vi "Main.vi"() -> ()   [LabVIEW 2021]
doc: "This template is for the Queued Message Handler design pattern.\n\nThe Event Handling Loop generates messages based on user interface actions.\n\nThe Message Handling Loop processes messages generated by the Event Handling Loop, or by other messages. The messages are string values, so new messages can be added easily to the Message Cases case structure in the Message Handling Loop. Each message cluster can also provide an optional value for Message Data, which is a variant that can be converted to whatever message-specific data is required."
uses:
  Controls/UI Data.ctl
  support/Message Queue/Message Queue.lvlib
  <vilib>/Utility/error.llb/Error Cluster From Error Code.vi
  support/User Event - Stop/User Event - Stop.lvlib
  support/Message Queue/Enqueue Message (Single).vi
  <vilib>/ErrorRing/Error Ring.xnode
  Controls/Status Lights.ctl
panel:
  in  "Start Pressure Logging":bool
  out "Speed Indicator":dbl
  in  "Release Brake":bool
  in  "Retract":bool
  out "Status":T1
  in  "Speed (v)":dbl(knob) scale=0.0..5.0
  out "Status":string
  in  "Extend":bool
  in  "Apply Brake":bool
  in  "Exit":bool
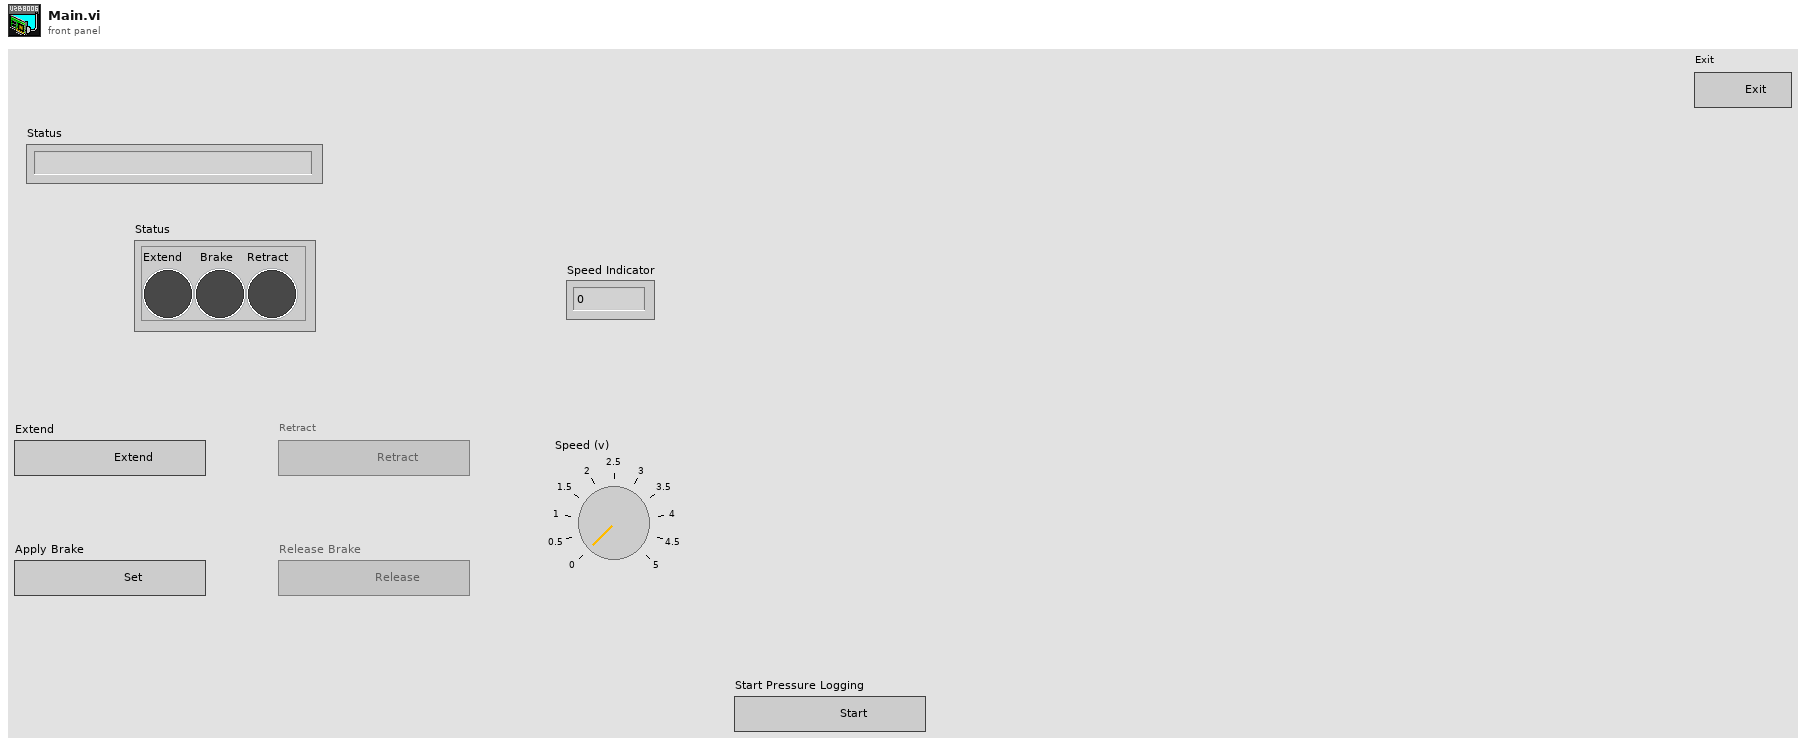
[diagram p1: front panel]
types:
  T1 = typedef "Status Lights.ctl" = cluster{"Extend":bool, "Brake":bool, "Retract":bool}
  T2 = typedef "UI Data.ctl" = cluster{"Boolean":bool, "String":string, "Speed":dbl, "Apply Brake Ref":refnum<vi>, "Release Brake Ref":refnum<vi>, "Extend Ref":refnum<vi>, "Retract Ref":refnum<vi>, "Data Display Ref":refnum<vi>, "Exit Button Ref":refnum<vi>, "Status":T1, "Pressure Ref":refnum<vi>}
  T3 = typedef "Message Queue.lvlib/All Message Queues.ctl" = cluster{"UI":refnum<queue>}
  T4 = typedef "DAQ Refnums.ctl" = cluster{"Direction Ref":refnum<k21>, "Brake Ref":refnum<k21>, "Speed Ref":refnum<k21>, "Pressure Ref":refnum<k21>}
  T5 = enum8{"Enabled", "Disabled", "Disabled and Grayed Out"}
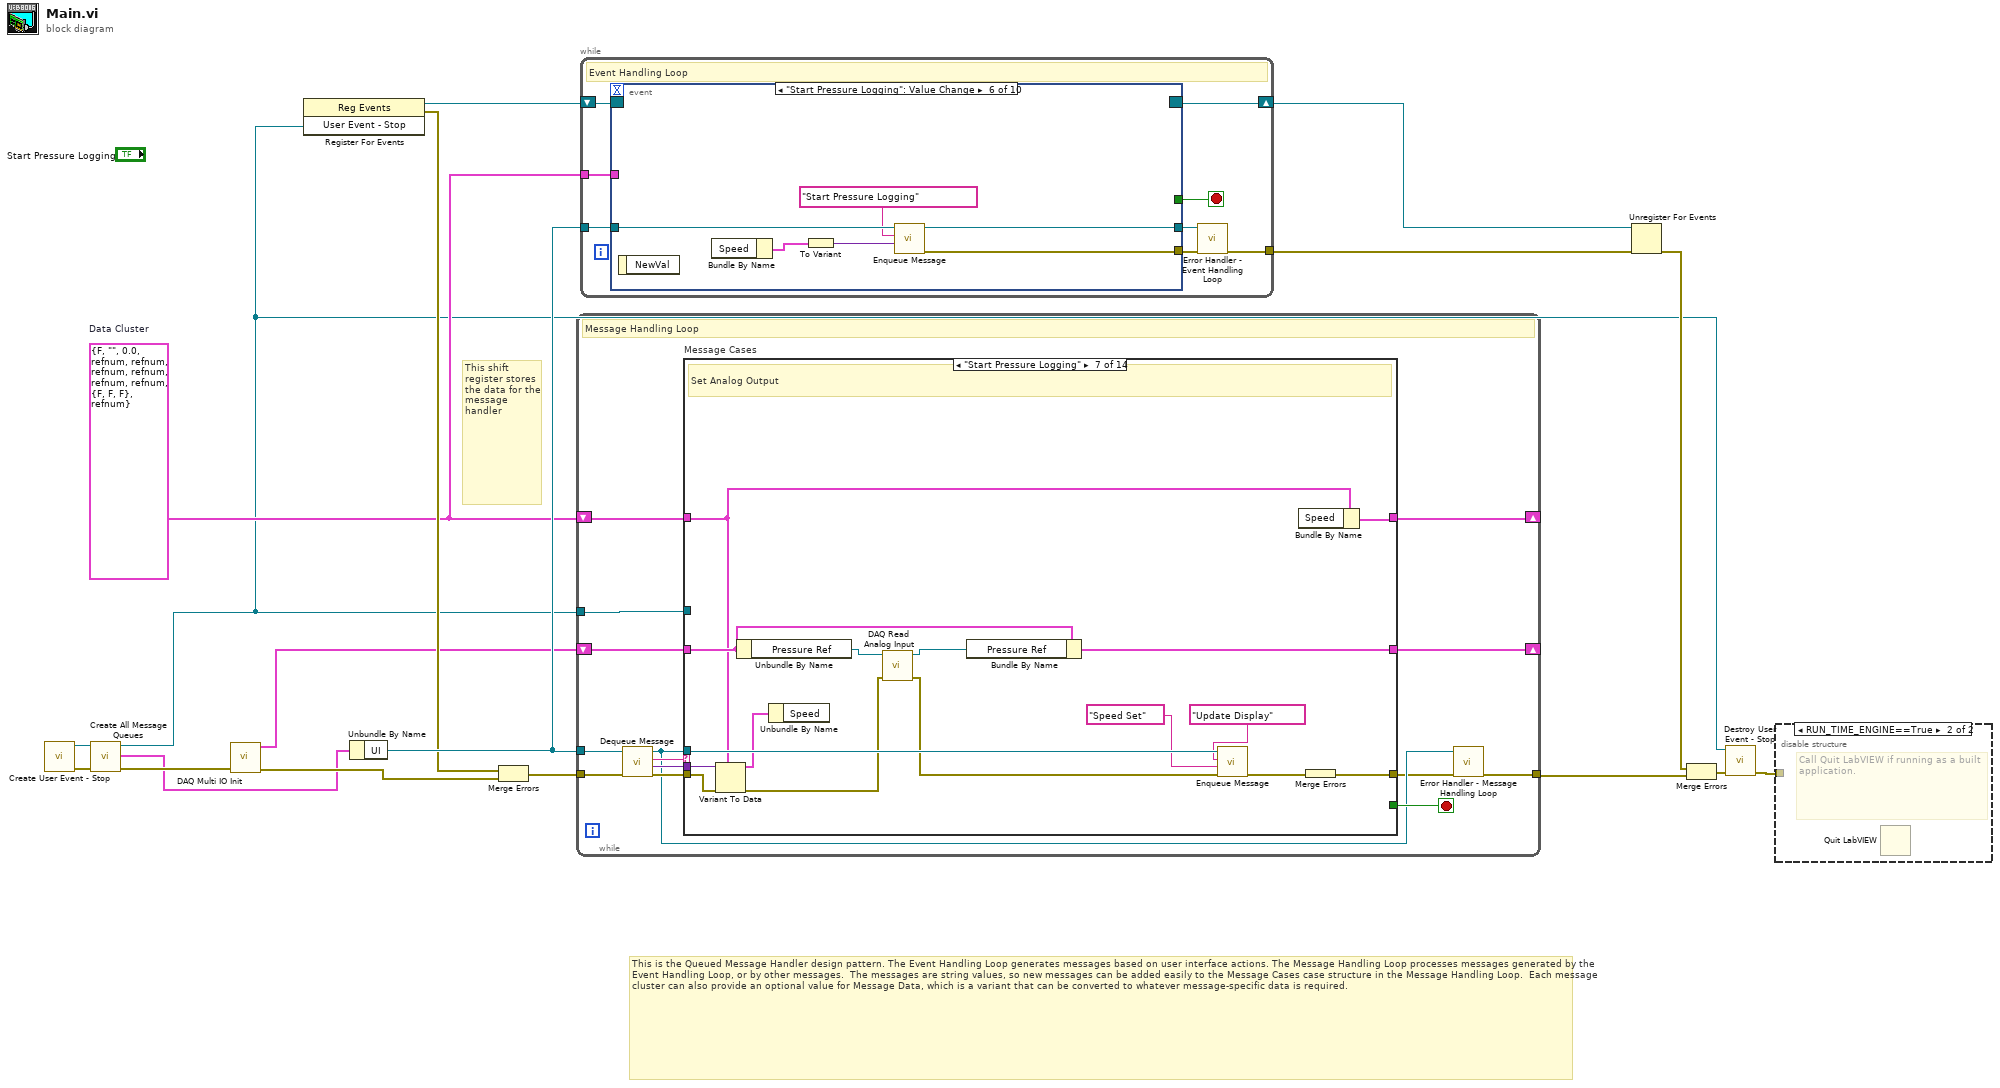
[diagram p0: block diagram]
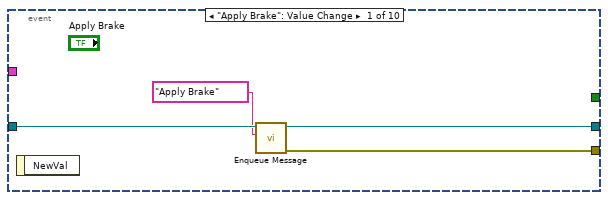
[diagram p3: hidden frame]
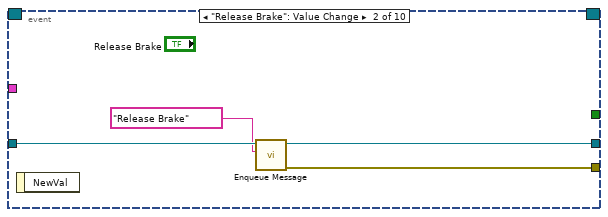
[diagram p4: hidden frame]
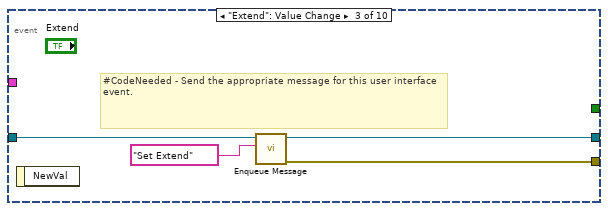
[diagram p5: hidden frame]
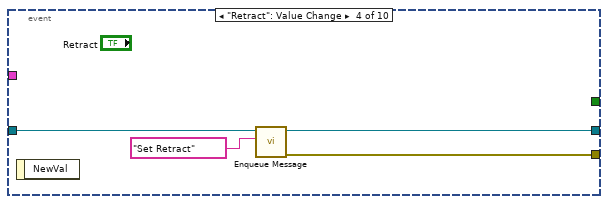
[diagram p6: hidden frame]
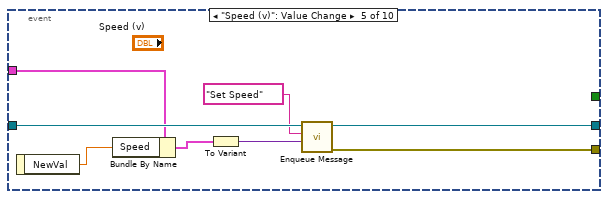
[diagram p7: hidden frame]
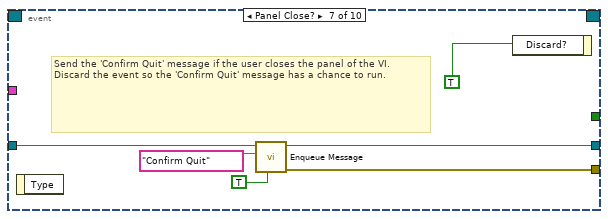
[diagram p8: hidden frame]
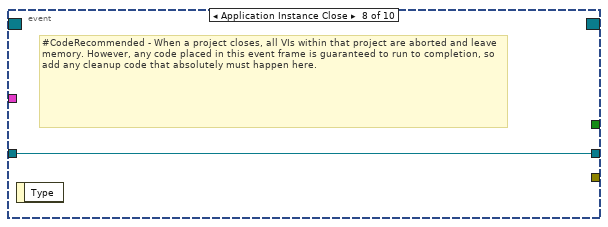
[diagram p9: hidden frame]
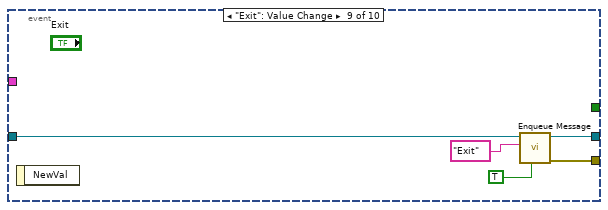
[diagram p10: hidden frame]
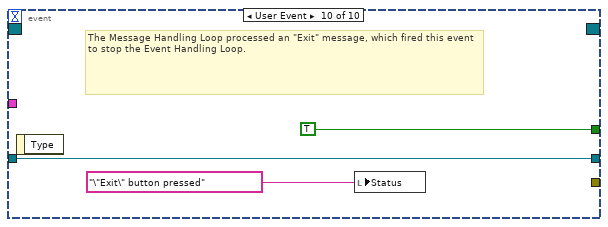
[diagram p11: hidden frame]
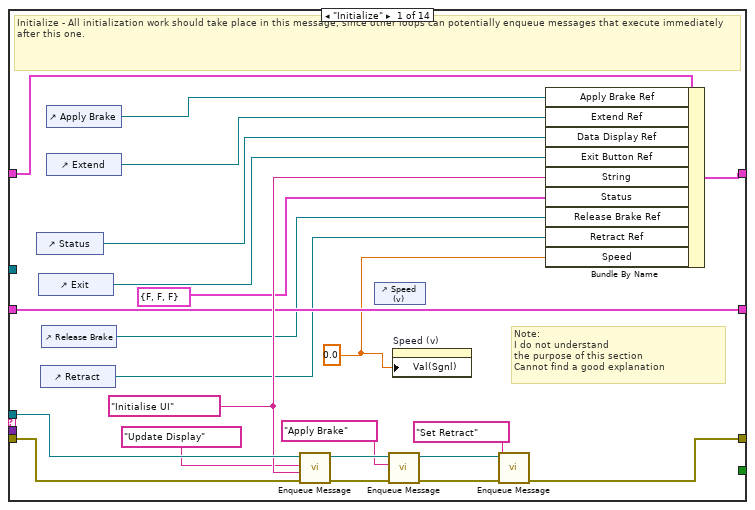
[diagram p12: hidden frame]
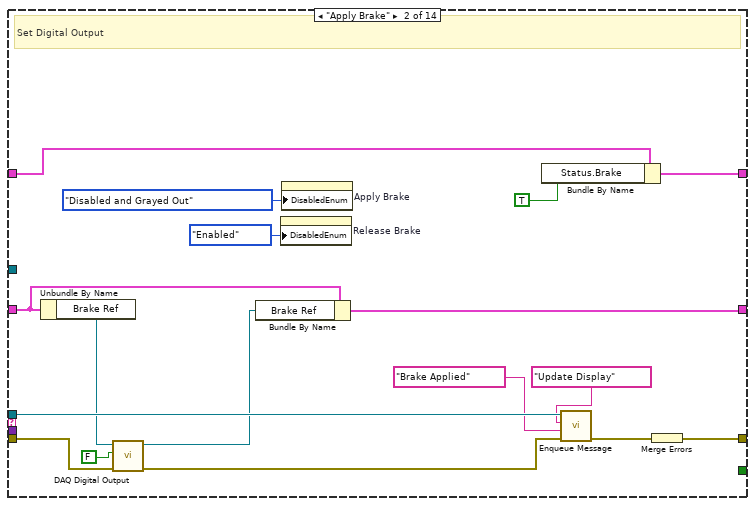
[diagram p13: hidden frame]
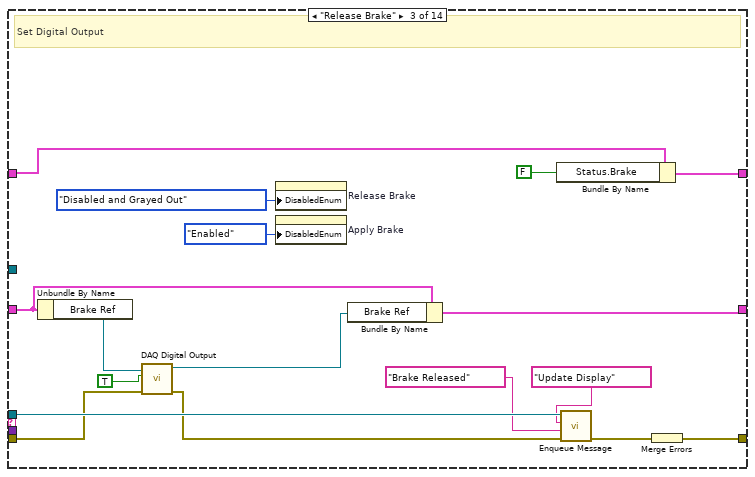
[diagram p14: hidden frame]
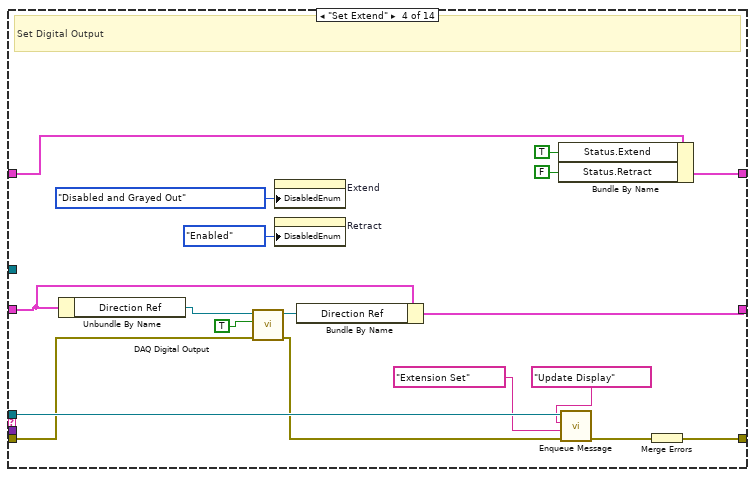
[diagram p15: hidden frame]
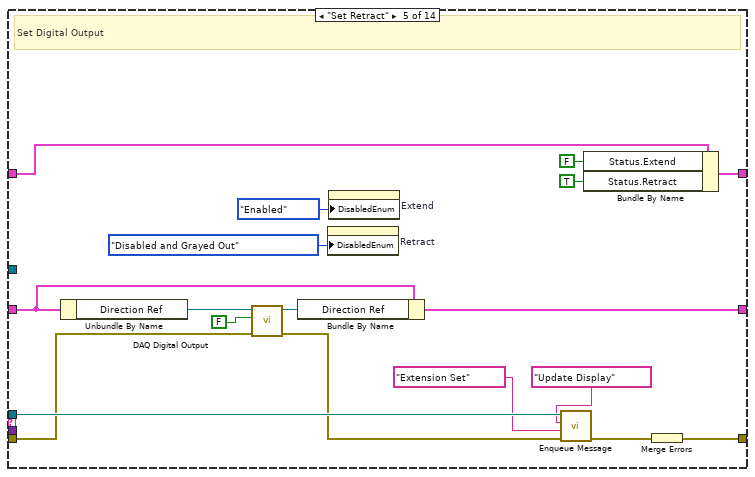
[diagram p16: hidden frame]
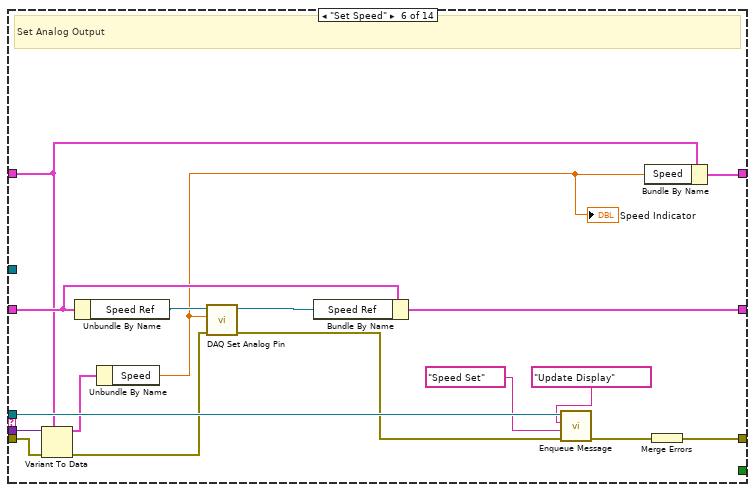
[diagram p17: hidden frame]
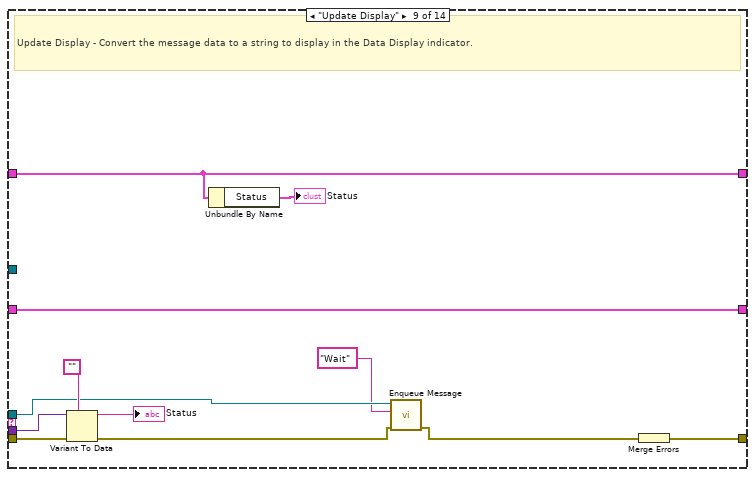
[diagram p19: hidden frame]
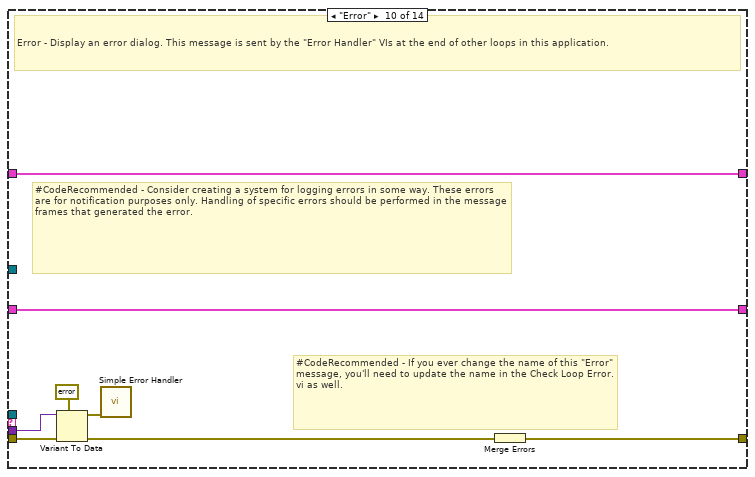
[diagram p20: hidden frame]
diagram:
  w5 = T2 {"Boolean"=FALSE, "String"="", "Speed"=0.0, "Apply Brake Ref"=refnum, "Release Brake Ref"=refnum, "Extend Ref"=refnum, "Retract Ref"=refnum, "Data Display Ref"=refnum, "Exit Button Ref"=refnum, "Status"={"Extend"=FALSE, "Brake"=FALSE, "Retract"=FALSE}, "Pressure Ref"=refnum}  # Data Cluster
  # "This is the Queued Message Handler design pattern. The Event Handling Loop generates messages based on user interface actions. The Message Handling Loop processes messages generated by the Event Handling Loop, or by other messages.  The messages are string values, so new messages can be added easily to the Message Cases case structure in the Message Handling Loop.  Each message cluster can also provide an optional value for Message Data, which is a variant that can be converted to whatever message-specific data is required."
  # "This shift register stores the data for the message handler"
  n1 = call "Create User Event - Stop.vi"() -> ("error out"=w16:errorcluster, "User Event - Stop"=w4:refnum<user-event>)  [unwired: 10 in]
  n2 = call "Create All Message Queues.vi"("error in (no error)"=w16) -> ("error out"=w3:errorcluster, "Message Queues out"=w1:T3)  [unwired: 9 in]
  n3 = call "DAQ Multi IO Init.vi"("error in"=w3) -> ("error out"=w2:errorcluster, "DAQ Ref Cluster"=w6:T4)  [unwired: 9 in]
  n4 = register-events(w4) -> (reference out=w10:refnum<event-registration>, error out=w9:errorcluster)  [unwired: 2 in]
  n5 = Unbundle By Name(w1) -> ("UI"=w17:refnum<queue>)
  n6 = Merge Errors(w9, w2) -> (w7:errorcluster)
  n7 = while {
    tunnel: w17 -> [w25]
    shift-right: [w20] -> _
    shift-left: w5 -> [w31]
    tunnel: w4 -> [w29]
    tunnel: [w23] -> w8
    tunnel: w7 -> [w21]
    shift-right: [w18] -> _
    shift-left: w6 -> [w19]
    stop <- w30 stop-if-true
    # "Message Handling Loop"
    n8 = call "Dequeue Message.vi"("error in (no error)"=w21, "Message Queue"=w25) -> ("error out"=w28:errorcluster, "Message Data"=w26:variant, "Message"=w27:string, "dup Message Queue"=w24:refnum<queue>)  [unwired: 6 in]
    n9 = case "Message Cases" shown="\"Start Pressure Logging\"" w27 {
      selector: w27 -> [_ _ _ _ _ _ _ _ _ _ _ _ _ w215]
      tunnel: w24 -> [w49 w68 w85 w103 w121 w138 w154 _ w162 _ w183 _ w213 _]
      tunnel: w28 -> [w53 w66 w83 w101 w119 w129 w148 w158 w170 w179 w187 w191 w208 _]
      tunnel: [w34 w70 w87 w105 w123 w140 w156 w158 w171 w173 w185 w189 w210 w216] -> w22
      tunnel: w31 -> [w41 w60 w71 w88 w108 w126 w146 w159 w166 w178 w186 w190 w212 w217]
      tunnel: [w52 w63 w80 w98 w116 w125 w145 w159 w166 w178 w186 w190 w212 w217] -> w20
      tunnel: [_ _ _ _ _ _ _ _ _ _ _ _ TRUE _] -> w30
      tunnel: w26 -> [_ _ _ _ _ w130 w149 _ w169 w177 _ _ w205 _]
      tunnel: w29 -> [_ _ _ _ _ _ _ _ _ _ _ _ w209 _]
      tunnel: w19 -> [w45 w58 w75 w94 w112 w135 w151 w157 w160 w172 w180 w188 w197 w214]
      tunnel: [w45 w57 w74 w93 w111 w134 w150 w157 w160 w172 w180 w188 w198 w214] -> w18
      frame "Initialize" {
        w42 = 0.0 ("Speed")
        w48 = "Initialise UI" ("Initial Message")
        # "Note:\nI do not understand\nthe purpose of this section\nCannot find a good explanation"
        # "Initialize - All initialization work should take place in this message, since other loops can potentially enqueue messages that execute immediately after this one."
        n10 = control-ref of="Status"() -> (w51:refnum<vi>)
        n11 = control-ref of="Exit"() -> (w50:refnum<vi>)
        n12 = control-ref of="Retract"() -> (w43:refnum<vi>)
        n13 = control-ref of="Release Brake"() -> (w44:refnum<vi>)
        n14 = control-ref of="Apply Brake"() -> (w47:refnum<vi>)
        n15 = control-ref of="Extend"() -> (w40:refnum<vi>)
        n16 = call-poly "Enqueue Message.vi"("error in (no error)"=w53, "Message Data"=w48, "Message"="Update Display", "Message Queue"=w49) -> ("error out"=w38:errorcluster, "dup Message Queue"=w37:refnum<queue>)  [unwired: 6 in]
        n17 = control-ref of="Speed (v)"() -> ()  [unwired: 1 out]
        n18 = call-poly "Enqueue Message.vi"("error in (no error)"=w38, "Message"="Apply Brake", "Message Queue"=w37) -> ("error out"=w35:errorcluster, "dup Message Queue"=w33:refnum<queue>)  [unwired: 7 in]
        n19 = property on="Speed (v)" class="Knob (strict)"("Val(Sgnl)"=w42) -> ()  [unwired: 2 in, 2 out]
        n20 = call-poly "Enqueue Message.vi"("error in (no error)"=w35, "Message"="Set Retract", "Message Queue"=w33) -> ("error out"=w34:errorcluster)  [unwired: 7 in, 1 out]
        n21 = Bundle By Name(cluster=w41, "Apply Brake Ref"=w47, "Extend Ref"=w40, "Data Display Ref"=w51, "Exit Button Ref"=w50, "String"=w48, "Status"=T1 {"Extend"=FALSE, "Brake"=FALSE, "Retract"=FALSE}, "Release Brake Ref"=w44, "Retract Ref"=w43, "Speed"=w42) -> (w52:T2)
      }
      frame "Apply Brake" {
        # "Set Digital Output"
        n22 = Unbundle By Name(w58) -> ("Brake Ref"=w59:refnum<k21>)
        n23 = call "DAQ Digital Output.vi"("error in"=w66, "data"=FALSE, "task/channels in"=w59) -> ("error out"=w65:errorcluster, "task out"=w56:refnum<k21>)  [unwired: 6 in, 1 out]
        n24 = Bundle By Name(cluster=w58, "Brake Ref"=w56) -> (w57:T4)
        n25 = property on="Release Brake" class="Bool"("DisabledEnum"=T5."Enabled" ("Disabled")) -> ()  [unwired: 2 in, 2 out]
        n26 = property on="Apply Brake" class="Bool"("DisabledEnum"=T5."Disabled and Grayed Out" ("Disabled")) -> ()  [unwired: 2 in, 2 out]
        n27 = Bundle By Name(cluster=w60, "Status.Brake"=TRUE) -> (w63:T2)
        n28 = call-poly "Enqueue Message.vi"("error in (no error)"=w65, "Message Data"="Brake Applied" ("\"Do Something\" button pressed"), "Message"="Update Display", "Message Queue"=w68) -> ("error out"=w69:errorcluster)  [unwired: 6 in, 1 out]
        n29 = Merge Errors(w69) -> (w70:errorcluster)
      }
      frame "Release Brake" {
        # "Set Digital Output"
        n30 = Unbundle By Name(w75) -> ("Brake Ref"=w77:refnum<k21>)
        n31 = call "DAQ Digital Output.vi"("error in"=w83, "data"=TRUE, "task/channels in"=w77) -> ("error out"=w82:errorcluster, "task out"=w76:refnum<k21>)  [unwired: 6 in, 1 out]
        n32 = property on="Release Brake" class="Bool"("DisabledEnum"=T5."Disabled and Grayed Out" ("Disabled")) -> ()  [unwired: 2 in, 2 out]
        n33 = property on="Apply Brake" class="Bool"("DisabledEnum"=T5."Enabled" ("Disabled")) -> ()  [unwired: 2 in, 2 out]
        n34 = Bundle By Name(cluster=w75, "Brake Ref"=w76) -> (w74:T4)
        n35 = Bundle By Name(cluster=w71, "Status.Brake"=FALSE ("Boolean")) -> (w80:T2)
        n36 = call-poly "Enqueue Message.vi"("error in (no error)"=w82, "Message Data"="Brake Released" ("\"Do Something\" button pressed"), "Message"="Update Display", "Message Queue"=w85) -> ("error out"=w86:errorcluster)  [unwired: 6 in, 1 out]
        n37 = Merge Errors(w86) -> (w87:errorcluster)
      }
      frame "Set Extend" {
        # "Set Digital Output"
        n38 = Unbundle By Name(w94) -> ("Direction Ref"=w96:refnum<k21>)
        n39 = call "DAQ Digital Output.vi"("error in"=w101, "data"=TRUE, "task/channels in"=w96) -> ("error out"=w100:errorcluster, "task out"=w95:refnum<k21>)  [unwired: 6 in, 1 out]
        n40 = property on="Extend" class="Bool"("DisabledEnum"=T5."Disabled and Grayed Out" ("Disabled")) -> ()  [unwired: 2 in, 2 out]
        n41 = property on="Retract" class="Bool"("DisabledEnum"=T5."Enabled" ("Disabled")) -> ()  [unwired: 2 in, 2 out]
        n42 = Bundle By Name(cluster=w94, "Direction Ref"=w95) -> (w93:T4)
        n43 = Bundle By Name(cluster=w88, "Status.Extend"=TRUE ("Status.Retract"), "Status.Retract"=FALSE ("Status.Extend")) -> (w98:T2)
        n44 = call-poly "Enqueue Message.vi"("error in (no error)"=w100, "Message Data"="Extension Set" ("\"Do Something\" button pressed"), "Message"="Update Display", "Message Queue"=w103) -> ("error out"=w104:errorcluster)  [unwired: 6 in, 1 out]
        n45 = Merge Errors(w104) -> (w105:errorcluster)
      }
      frame "Set Retract" {
        # "Set Digital Output"
        n46 = Unbundle By Name(w112) -> ("Direction Ref"=w114:refnum<k21>)
        n47 = call "DAQ Digital Output.vi"("error in"=w119, "data"=FALSE, "task/channels in"=w114) -> ("error out"=w118:errorcluster, "task out"=w113:refnum<k21>)  [unwired: 6 in, 1 out]
        n48 = Bundle By Name(cluster=w112, "Direction Ref"=w113) -> (w111:T4)
        n49 = property on="Retract" class="Bool"("DisabledEnum"=T5."Disabled and Grayed Out" ("Disabled")) -> ()  [unwired: 2 in, 2 out]
        n50 = property on="Extend" class="Bool"("DisabledEnum"=T5."Enabled" ("Disabled")) -> ()  [unwired: 2 in, 2 out]
        n51 = call-poly "Enqueue Message.vi"("error in (no error)"=w118, "Message Data"="Extension Set" ("\"Do Something\" button pressed"), "Message"="Update Display", "Message Queue"=w121) -> ("error out"=w122:errorcluster)  [unwired: 6 in, 1 out]
        n52 = Bundle By Name(cluster=w108, "Status.Extend"=FALSE ("Status.Retract"), "Status.Retract"=TRUE ("Status.Extend")) -> (w116:T2)
        n53 = Merge Errors(w122) -> (w123:errorcluster)
      }
      frame "Set Speed" {
        # "Set Analog Output"
        n54 = Variant To Data(error in=w129, type=w126, Variant=w130) -> (data=w127:T2, error out=w128:errorcluster)
        n55 = Unbundle By Name(w135) -> ("Speed Ref"=w133:refnum<k21>)
        n56 = Unbundle By Name(w127) -> ("Speed"=w124:dbl)
        "Speed Indicator" <- w124
        n57 = call "DAQ Set Analog Pin.vi"("error in"=w128, "Voltage"=w124, "task/channels in"=w133) -> ("error out"=w131:errorcluster, "task out"=w132:refnum<k21>)  [unwired: 6 in, 1 out]
        n58 = Bundle By Name(cluster=w135, "Speed Ref"=w132) -> (w134:T4)
        n59 = call-poly "Enqueue Message.vi"("error in (no error)"=w131, "Message Data"="Speed Set" ("\"Do Something\" button pressed"), "Message"="Update Display", "Message Queue"=w138) -> ("error out"=w139:errorcluster)  [unwired: 6 in, 1 out]
        n60 = Bundle By Name(cluster=w126, "Speed"=w124) -> (w125:T2)
        n61 = Merge Errors(w139) -> (w140:errorcluster)
      }
      frame "Start Pressure Logging" {
        # "Set Analog Output"
        n62 = Variant To Data(error in=w148, type=w146, Variant=w149) -> (data=w147:T2, error out=w143:errorcluster)
        n63 = Unbundle By Name(w151) -> ("Pressure Ref"=w144:refnum<k21>)
        n64 = Unbundle By Name(w147) -> ()  [unwired: 1 out]
        n65 = call "DAQ Read Analog Input.vi"("error in"=w143, "task/channels in"=w144) -> ("error out"=w142:errorcluster, "task out"=w141:refnum<k21>)  [unwired: 7 in, 1 out]
        n66 = Bundle By Name(cluster=w151, "Pressure Ref"=w141) -> (w150:T4)
        n67 = call-poly "Enqueue Message.vi"("error in (no error)"=w142, "Message Data"="Speed Set" ("\"Do Something\" button pressed"), "Message"="Update Display", "Message Queue"=w154) -> ("error out"=w155:errorcluster)  [unwired: 6 in, 1 out]
        n68 = Bundle By Name(cluster=w146) -> (w145:T2)  [unwired: 1 in]
        n69 = Merge Errors(w155) -> (w156:errorcluster)
      }
      frame "Wait" {
        # "Wait case - wait for user input"
      }
      frame "Update Display" {
        # "Update Display - Convert the message data to a string to display in the Data Display indicator."
        n70 = Variant To Data(error in=w170, type="", Variant=w169) -> (data=→"Status":string, error out=w164:errorcluster)
        n71 = Unbundle By Name(w166) -> ("Status"=→"Status":T1)
        n72 = call-poly "Enqueue Message.vi"("error in (no error)"=w164, "Message"="Wait", "Message Queue"=w162) -> ("error out"=w163:errorcluster)  [unwired: 7 in, 1 out]
        n73 = Merge Errors(w163) -> (w171:errorcluster)
      }
      frame "Error" {
        # "#CodeRecommended - If you ever change the name of this \"Error\" message, you'll need to update the name in the Check Loop Error.vi as well."
        # "#CodeRecommended - Consider creating a system for logging errors in some way. These errors are for notification purposes only. Handling of specific errors should be performed in the message frames that generated the error."
        # "Error - Display an error dialog. This message is sent by the \"Error Handler\" VIs at the end of other loops in this application."
        n74 = Variant To Data(error in=w179, type=errorcluster {"status"=FALSE, "code"=0, "source"=""} ("error constant"), Variant=w177) -> (data=w175:errorcluster, error out=w174:errorcluster)
        n75 = call <vilib>:"Simple Error Handler.vi"("error in (no error)"=w175) -> ()  [unwired: 4 in, 5 out]
        n76 = Merge Errors(w174) -> (w173:errorcluster)
      }
      frame "Confirm Quit" {
        # "#CodeNeeded - If you want to provide an \"Are you sure\" dialog (or some other notification) before the application exits, place that code here. This message is typically sent from a Panel Close? event."
        # "Confirm Quit - Message that can confirm whether or not the user wants to exit the application."
        n77 = call-poly "Enqueue Message.vi"("Priority Message? (F)"=TRUE, "error in (no error)"=w187, "Message"="Exit", "Message Queue"=w183) -> ("error out"=w184:errorcluster)  [unwired: 6 in, 1 out]
        n78 = Merge Errors(w184) -> (w185:errorcluster)
      }
      frame "---Copy This Frame---" {
        # "Duplicate this frame when creating new messages.  Change this comment in the duplicated frame to describe this message."
        n79 = Merge Errors(w191) -> (w189:errorcluster)
      }
      frame "Exit" {
        # "Stop the VI"
        # "Release the message queue reference"
        # "Exit - Exit the application."
        n80 = Release Queue(queue=w213, error in (no error)=w208) -> (error out=w204:errorcluster)  [unwired: 1 in, 2 out]
        n81 = call "Fire User Event - Stop.vi"("User Event - Stop"=w209) -> ("error out"=w193:errorcluster)  [unwired: 10 in]
        n82 = Variant To Data(type=errorcluster {"status"=FALSE, "code"=0, "source"=""} ("error constant"), Variant=w205) -> (data=w206:errorcluster)  [unwired: 1 in, 1 out]
        n83 = Unbundle By Name(w197) -> ("Direction Ref"=w201:refnum<k21>, "Brake Ref"=w200:refnum<k21>, "Speed Ref"=w199:refnum<k21>)
        n84 = call <vilib>:"Simple Error Handler.vi"("error in (no error)"=w206) -> ()  [unwired: 4 in, 5 out]
        n85 = call <vilib>:"DAQmx Clear Task.vi"("task in"=w199, "error in"=w204) -> ("error out"=w203:errorcluster)  [unwired: 13 in]
        n86 = call <vilib>:"DAQmx Clear Task.vi"("task in"=w200, "error in"=w203) -> ("error out"=w202:errorcluster)  [unwired: 13 in]
        n87 = call <vilib>:"DAQmx Clear Task.vi"("task in"=w201, "error in"=w202) -> ("error out"=w192:errorcluster)  [unwired: 13 in]
        n88 = Bundle By Name(cluster=w197, "Direction Ref"=refnum<k21> refnum, "Brake Ref"=refnum<k21> refnum, "Speed Ref"=refnum<k21> refnum) -> (w198:T4)
        n89 = Merge Errors(w193, w192) -> (w210:errorcluster)
      }
      frame Default {
        # "'Default' case only runs if there is a message that isn't defined in any of the other cases.  Output a programming error."
        n90 = xnode "Error Ring"("parameter 0"=w215) -> ("error out"=w216:errorcluster)
      }
    }
    n91 = call "Error Handler - Message Handling Loop.vi"("error in (no error)"=w22, "Message Queue"=w24) -> ("dup error in"=w23:errorcluster)  [unwired: 8 in, 1 out]
  }
  n92 = while {
    tunnel: w17 -> [w232]
    shift-right: [w230] -> w13
    shift-left: w10 -> [w231]
    tunnel: [w226] -> w11
    tunnel: w5 -> [w225]
    stop <- w228 stop-if-true
    # "Event Handling Loop"
    n93 = event shown="[5] \"Start Pressure Logging\": Value Change" {
      selector: w231 -> [_ _ _ _ _ _ _ _ _ _]
      dyn-events: [_ _ _ _ _ _ _ _ _ _] -> w230
      timeout: _ -> [_ _ _ _ _ _ _ _ _ _]
      tunnel: [_ _ _ _ _ _ _ _ _ TRUE ("Discard?")] -> w228
      tunnel: w232 -> [w236 w240 w244 w248 w256 w262 w267 w269 w274 w277]
      tunnel: [w233 w237 w241 w245 w253 w259 w266 _ w273 _] -> w229
      tunnel: [w235 w239 w243 w247 w255 w261 w265 w269 w272 w277] -> w227
      tunnel: w225 -> [_ _ _ _ w249 _ _ _ _ _]
      event "Apply Brake": Value Change {
        n94 = event-data() -> ()  [unwired: 1 in, 1 out]
        n95 = call-poly "Enqueue Message.vi"("Message"="Apply Brake", "Message Queue"=w236) -> ("error out"=w233:errorcluster, "dup Message Queue"=w235:refnum<queue>)  [unwired: 8 in]
      }
      event "Release Brake": Value Change {
        n96 = event-data() -> ()  [unwired: 1 in, 1 out]
        n97 = call-poly "Enqueue Message.vi"("Message"="Release Brake", "Message Queue"=w240) -> ("error out"=w237:errorcluster, "dup Message Queue"=w239:refnum<queue>)  [unwired: 8 in]
      }
      event "Extend": Value Change {
        # "#CodeNeeded - Send the appropriate message for this user interface event."
        n98 = event-data() -> ()  [unwired: 1 in, 1 out]
        n99 = call-poly "Enqueue Message.vi"("Message"="Set Extend", "Message Queue"=w244) -> ("error out"=w241:errorcluster, "dup Message Queue"=w243:refnum<queue>)  [unwired: 8 in]
      }
      event "Retract": Value Change {
        n100 = event-data() -> ()  [unwired: 1 in, 1 out]
        n101 = call-poly "Enqueue Message.vi"("Message"="Set Retract", "Message Queue"=w248) -> ("error out"=w245:errorcluster, "dup Message Queue"=w247:refnum<queue>)  [unwired: 8 in]
      }
      event "Speed (v)": Value Change {
        n102 = event-data() -> ("NewVal"=w251:dbl)  [unwired: 1 in]
        n103 = Bundle By Name(cluster=w249, "Speed"=w251) -> (w250:T2)
        n104 = To Variant(anything=w250) -> (Variant=w252:variant)
        n105 = call-poly "Enqueue Message.vi"("Message Data"=w252, "Message"="Set Speed", "Message Queue"=w256) -> ("error out"=w253:errorcluster, "dup Message Queue"=w255:refnum<queue>)  [unwired: 7 in]
      }
      event "Start Pressure Logging": Value Change {
        n106 = event-data() -> ()  [unwired: 1 in, 1 out]
        n107 = Bundle By Name() -> (w257:cluster{})  [unwired: 2 in]
        n108 = To Variant(anything=w257) -> (Variant=w258:variant)
        n109 = call-poly "Enqueue Message.vi"("Message Data"=w258, "Message"="Start Pressure Logging", "Message Queue"=w262) -> ("error out"=w259:errorcluster, "dup Message Queue"=w261:refnum<queue>)  [unwired: 7 in]
      }
      event Panel Close? {
        # "Send the 'Confirm Quit' message if the user closes the panel of the VI. Discard the event so the 'Confirm Quit' message has a chance to run."
        n110 = event-data() -> ()  [unwired: 1 in, 1 out]
        n111 = call-poly "Enqueue Message.vi"("Priority Message? (F)"=TRUE, "Message"="Confirm Quit", "Message Queue"=w267) -> ("error out"=w266:errorcluster, "dup Message Queue"=w265:refnum<queue>)  [unwired: 7 in]
        n112 = event-data("Discard?"=TRUE) -> ()  [unwired: 1 in, 1 out]
      }
      event Application Instance Close {
        # "#CodeRecommended - When a project closes, all VIs within that project are aborted and leave memory. However, any code placed in this event frame is guaranteed to run to completion, so add any cleanup code that absolutely must happen here."
        n113 = event-data() -> ()  [unwired: 1 in, 1 out]
      }
      event "Exit": Value Change {
        n114 = event-data() -> ()  [unwired: 1 in, 1 out]
        n115 = call-poly "Enqueue Message.vi"("Priority Message? (F)"=TRUE, "Message"="Exit", "Message Queue"=w274) -> ("error out"=w273:errorcluster, "dup Message Queue"=w272:refnum<queue>)  [unwired: 7 in]
      }
      event User Event {
        # "The Message Handling Loop processed an \"Exit\" message, which fired this event to stop the Event Handling Loop."
        n116 = event-data() -> ()  [unwired: 1 in, 1 out]
        n117 = local write "Status"("\"Exit\" button pressed" ("VI Stopped")) -> ()
      }
    }
    n118 = call "Error Handler - Event Handling Loop.vi"("error in (no error)"=w229, "Message Queue"=w227) -> ("dup error in"=w226:errorcluster)  [unwired: 8 in, 1 out]
  }
  n119 = Unregister For Events(event registration refnum=w13, error in=w11) -> (error out=w14:errorcluster)
  n120 = Merge Errors(w14, w8) -> (w15:errorcluster)
  n121 = call "Destroy User Event - Stop.vi"("error in (no error)"=w15, "User Event - Stop"=w4) -> ("error out"=w12:errorcluster)  [unwired: 9 in]
  n122 = disable-structure shown="RUN_TIME_ENGINE==True" {
    disable-tunnel: w12 -> [_ _]
    frame condition #0 (active) {
    }
    frame condition #1 {
      # "Call Quit LabVIEW if running as a built application."
      n123 = Quit LabVIEW() -> ()  [unwired: 1 in]
    }
  }
